vi "Calibrate Gripper.vi"(2 "node":string, 3 "Side":T1, 6 "error in":errorcluster) -> (5 "error out":errorcluster)   [LabVIEW 2013]
doc: "Calibrate the left or right gripper"
uses:
  ROS/Code/SubVIs/BaxterSide.ctl
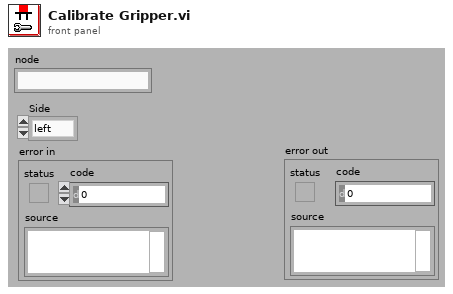
[diagram p1: front panel]
types:
  T1 = typedef "BaxterSide.ctl" = enum16{"left", "right"}
  T2 = typedef "_ROSControl.ctl" = cluster{"topic port":u16, "Node":string, "topic":string, "type":string, "node port":u32, "error ":errorcluster, "Direction":T3, "APIs":string[]}
  T3 = typedef "_ROSDirection.ctl" = enum16{"Node", "Publisher", "Subscriber", "Service Client"}
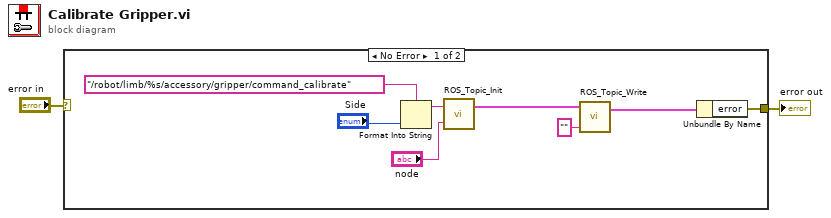
[diagram p0: block diagram]
diagram:
  n1 = case shown="No Error" "error in" {
    selector: "error in" -> [_ w11]
    tunnel: [w8 w11] -> w2
    frame No Error {
      n2 = Format Into String(format string="/robot/limb/%s/accessory/gripper/command_calibrate" ("topic"), "Side") -> (resulting string=w5:string)  [unwired: 2 in, 1 out]
      n3 = call "ROS_Topic_Init.vi"("node"="node", "topic"=w5) -> ("ROS out"=w10:T2)  [unwired: 1 in]
      n4 = call "ROS_Topic_Write.vi"("Msg in"="" ("Empty Command"), "ROS in"=w10) -> ("ROS out"=w9:T2)  [unwired: 2 in]
      n5 = Unbundle By Name(w9) -> ("error"=w8:errorcluster)
    }
    frame Error {
    }
  }
  "error out" <- w2
